vi "Rsync Log Files to Server.vi"(6 "System Net Name":string, 7 "Recipients":string="controlroom@magnet.fsu.edu", 8 "Error In":errorcluster, 9 "Log File Template":string, 11 "Log File Path In":path) -> (0 "Error Out":errorcluster, 1 "Standard Output":string, 2 "Return Code":i32, 3 "Log File Path Out":path, 4 "Standard Error":string)   [LabVIEW 2021]
uses:
  RT Host Globals.vi
panel:
  out "Send Mail Error Out":errorcluster={"status"=FALSE, "code"=1, "source"=""}
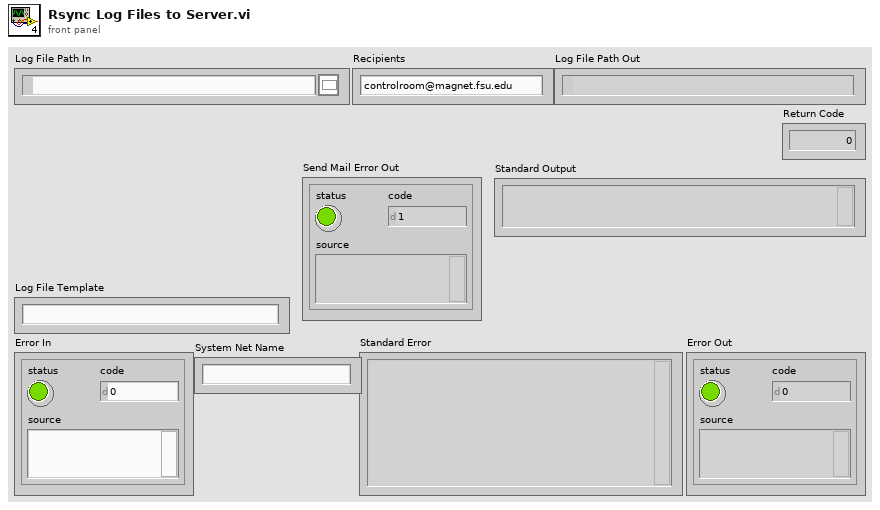
[diagram p1: front panel]
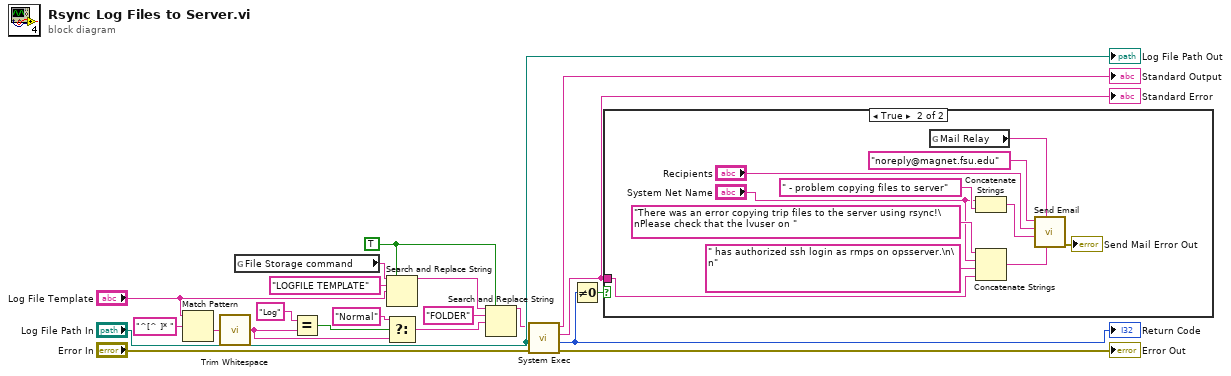
[diagram p0: block diagram]
diagram:
  w9 = TRUE ("replace all? (F)")
  n1 = Match Pattern(string="Log File Template", regular expression="^[^ ]* ") -> (after substring=w11:string)  [unwired: 1 in, 3 out]
  n2 = call <vilib>:"Trim Whitespace.vi"("string"=w11) -> ("trimmed string"=w3:string)  [unwired: 1 in]
  n3 = global read "RT Host Globals.vi" "File Storage command"() -> (w1:string)
  n4 = Equal?(x="Log" ("y"), y=w3) -> (x = y?=w6:bool)
  n5 = Search and Replace String(replace all?=w9, input string=w1, search string="LOGFILE TEMPLATE", replace string="Log File Template") -> (result string=w8:string)  [unwired: 4 in, 3 out]
  n6 = Select(t="Normal", s=w6, f=w3) -> (s? t:f=w5:string)
  n7 = Search and Replace String(replace all?=w9, input string=w8, search string="FOLDER", replace string=w5) -> (result string=w7:string)  [unwired: 4 in, 3 out]
  n8 = call <vilib>:"System Exec.vi"("error in (no error)"="Error In", "working directory"="Log File Path In", "command line"=w7) -> ("error out"=→"Error Out":errorcluster, "return code"=w15:i32, "standard error"=w14:string, "standard output"=→"Standard Output":string)  [unwired: 5 in]
  "Standard Error" <- w14
  "Return Code" <- w15
  n9 = Not Equal To 0?(x=w15) -> (x != 0?=w16:bool)
  n10 = case shown="True" w16 {
    tunnel: w14 -> [_ w30]
    frame False {
    }
    frame True {
      n11 = global read "RT Host Globals.vi" "Mail Relay"() -> (w22:string)
      n12 = Concatenate Strings("System Net Name", " - problem copying files to server" ("Subject")) -> (w29:string)
      n13 = Concatenate Strings("There was an error copying trip files to the server using rsync!\nPlease check that the lvuser on " ("string"), "System Net Name", " has authorized ssh login as rmps on opsserver.\n\n" ("Message"), w30) -> (w24:string)
      n14 = call "Send Email.vi"("Message"=w24, "Server Address"=w22, "Subject"=w29, "Recipients"="Recipients", "From"="noreply@magnet.fsu.edu" ("from")) -> ("error out"=→"Send Mail Error Out":errorcluster)  [unwired: 6 in]
    }
  }
  "Log File Path Out" <- "Log File Path In"
